vi "populate_list.vi"(7 "selected item (index)":i32, 8 "error in (no error)":errorcluster, 10 "steps":T1[](array[typedef]), 11 "list ctrl reference":refnum<vi>) -> (0 "error out":errorcluster)   [LabVIEW 2010]
uses:
  common/clusters/plugin_specification.ctl
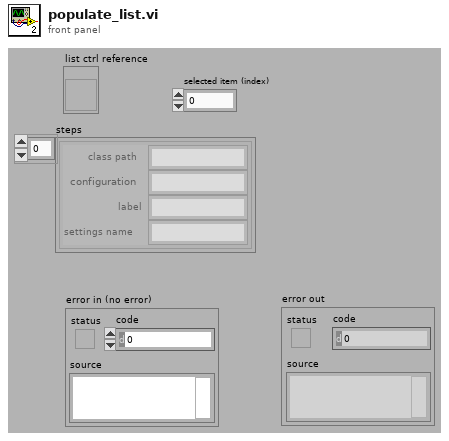
[diagram p1: front panel]
types:
  T1 = typedef "plugin_specification.ctl" = cluster{"class path":string, "configuration":string, "label":string, "settings name":string}
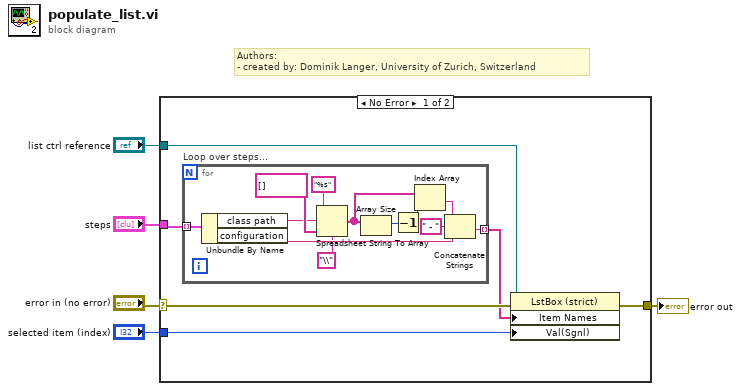
[diagram p0: block diagram]
diagram:
  # "Authors: \n- created by: Dominik Langer, University of Zurich, Switzerland"
  n1 = case shown="No Error" "error in (no error)" {
    selector: "error in (no error)" -> [w9 w23]
    tunnel: "steps" -> [w10 _]
    tunnel: [w9 w23] -> w3
    tunnel: "list ctrl reference" -> [w7 _]
    tunnel: "selected item (index)" -> [w6 _]
    frame No Error {
      n2 = for "Loop over steps..." {
        tunnel: w10 -> [w22] mode=indexing
        tunnel: [w19] -> w8 mode=indexing
        n3 = Unbundle By Name(w22) -> ("class path"=w16:string, "configuration"=w21:string)
        n4 = Spreadsheet String To Array(delimiter (Tab)="\\" ("search string/char (-)"), format string="%s", spreadsheet string=w16, array type (2D Dbl)=string[] []) -> (array=w15:string[])
        n5 = Array Size(array=w15) -> (size(s)=w13:i32)
        n6 = Decrement(x=w13) -> (x-1=w12:i32)
        n7 = Index Array(array=w15, index=w12) -> (element=w14:string)
        n8 = Concatenate Strings(w14, " - " ("string"), w21) -> (w19:string)
      }
      n9 = property on="Property Node" class="LstBox (strict)"(reference=w7, error in=w9, "Item Names"=w8, "Val(Sgnl)"=w6) -> ()  [unwired: 2 out]
    }
    frame Error {
    }
  }
  "error out" <- w3
